vi "fetchBTFData_chaos.vi"(0 "Funcion":u16(ring) items=["Init", "Run", "Close"], 1 "!CHAOS WAN url":u32=10000) -> (3 "lastTrigger":i32, 4 "Array":i32[](array[numeric]), 5 "# of elements":i32, 6 "ReadError":bool, 7 "DataReady":bool)   [LabVIEW 2014]
panel:
  # "Version:\n- 1.0 UDP to MC\n- 1.1 deduce dataready \n\nto be done:\n- manage errori"
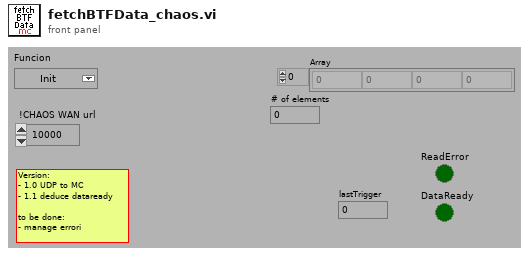
[diagram p1: front panel]
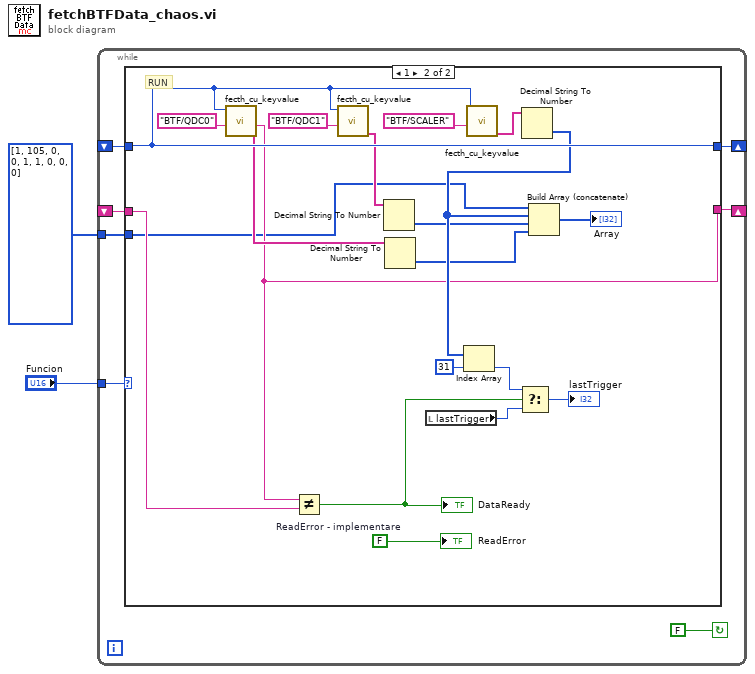
[diagram p0: block diagram]
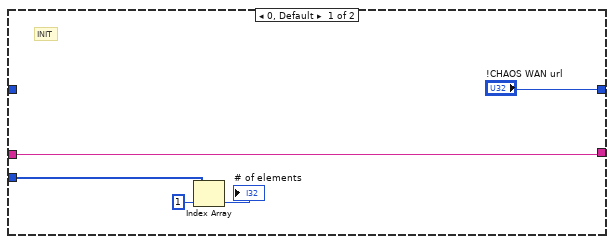
[diagram p2: hidden frame]
diagram:
  n1 = while {
    shift-left: _ -> [w8]
    shift-right: [w7] -> _
    tunnel: "Funcion" -> [w9]
    shift-right: [w5] -> _
    shift-left: _ -> [w4]
    tunnel: i32[] [1, 105, 0, 0, 1, 1, 0, 0, 0] -> [w3]
    stop <- FALSE continue-if-true
    n2 = case shown="1" w9 {
      tunnel: w8 -> [_ w25]
      tunnel: ["!CHAOS WAN url" w25] -> w7
      tunnel: [w13 w18] -> w5
      tunnel: w4 -> [w13 w31]
      tunnel: w3 -> [w12 w17]
      frame 0, Default {
        # "INIT"
        n3 = Index Array(array=w12, index=1) -> (element=→"# of elements":i32)
      }
      frame 1 {
        w29 = FALSE  # ReadError - implementare
        # "RUN"
        n4 = call "fecth_cu_keyvalue.vi"("cuname"="BTF/QDC0", "handleConnection"=w25) -> ("data out"=w19:string[], "timestemp"=w18:string)  [unwired: 4 in, 4 out]
        n5 = Not Equal?(x=w18, y=w31) -> (x != y?=w30:bool)
        "DataReady" <- w30
        n6 = call "fecth_cu_keyvalue.vi"("cuname"="BTF/QDC1", "handleConnection"=w25) -> ("data out"=w20:string[])  [unwired: 4 in, 5 out]
        n7 = Decimal String To Number(string=w20) -> (number=w16:i32[])  [unwired: 2 in, 1 out]
        n8 = Decimal String To Number(string=w19) -> (number=w15:i32[])  [unwired: 2 in, 1 out]
        n9 = local read "lastTrigger"() -> (w32:i32)
        n10 = call "fecth_cu_keyvalue.vi"("cuname"="BTF/SCALER", "handleConnection"=w25) -> ("data out"=w23:string[])  [unwired: 4 in, 5 out]
        n11 = Decimal String To Number(string=w23) -> (number=w22:i32[])  [unwired: 2 in, 1 out]
        n12 = Index Array(array=w22, index=31) -> (element=w33:i32)
        n13 = Select(t=w33, s=w30, f=w32) -> (s? t:f=→"lastTrigger":i32)
        n14 = Build Array (concatenate)(w17, w22, w16, w15) -> (→"Array":i32[])
        "ReadError" <- w29
      }
    }
  }
